vi "DerotatorControl_byYaw.vi"() -> ()   [LabVIEW 2021]
uses:
  <vilib>/DAQmx/write.llb/DAQmx Write (Digital Bool 1Line 1Point).vi
  <vilib>/DAQmx/create/channels.llb/DAQmx Create Channel (DO-Digital Output).vi
  <vilib>/DAQmx/miscellaneous.llb/DAQmx Fill In Error Info.vi
  GlobalYAW.vi
panel:
  out "Pitch":dbl(slide) scale=-90.0..90.0
  out "Roll":dbl(slide) scale=-180.0..180.0
  out "Yaw":dbl(slide) scale=-180.0..180.0
  in  "stop":bool
  in  "Record!":bool
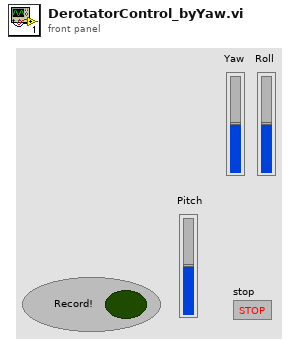
[diagram p1: front panel]
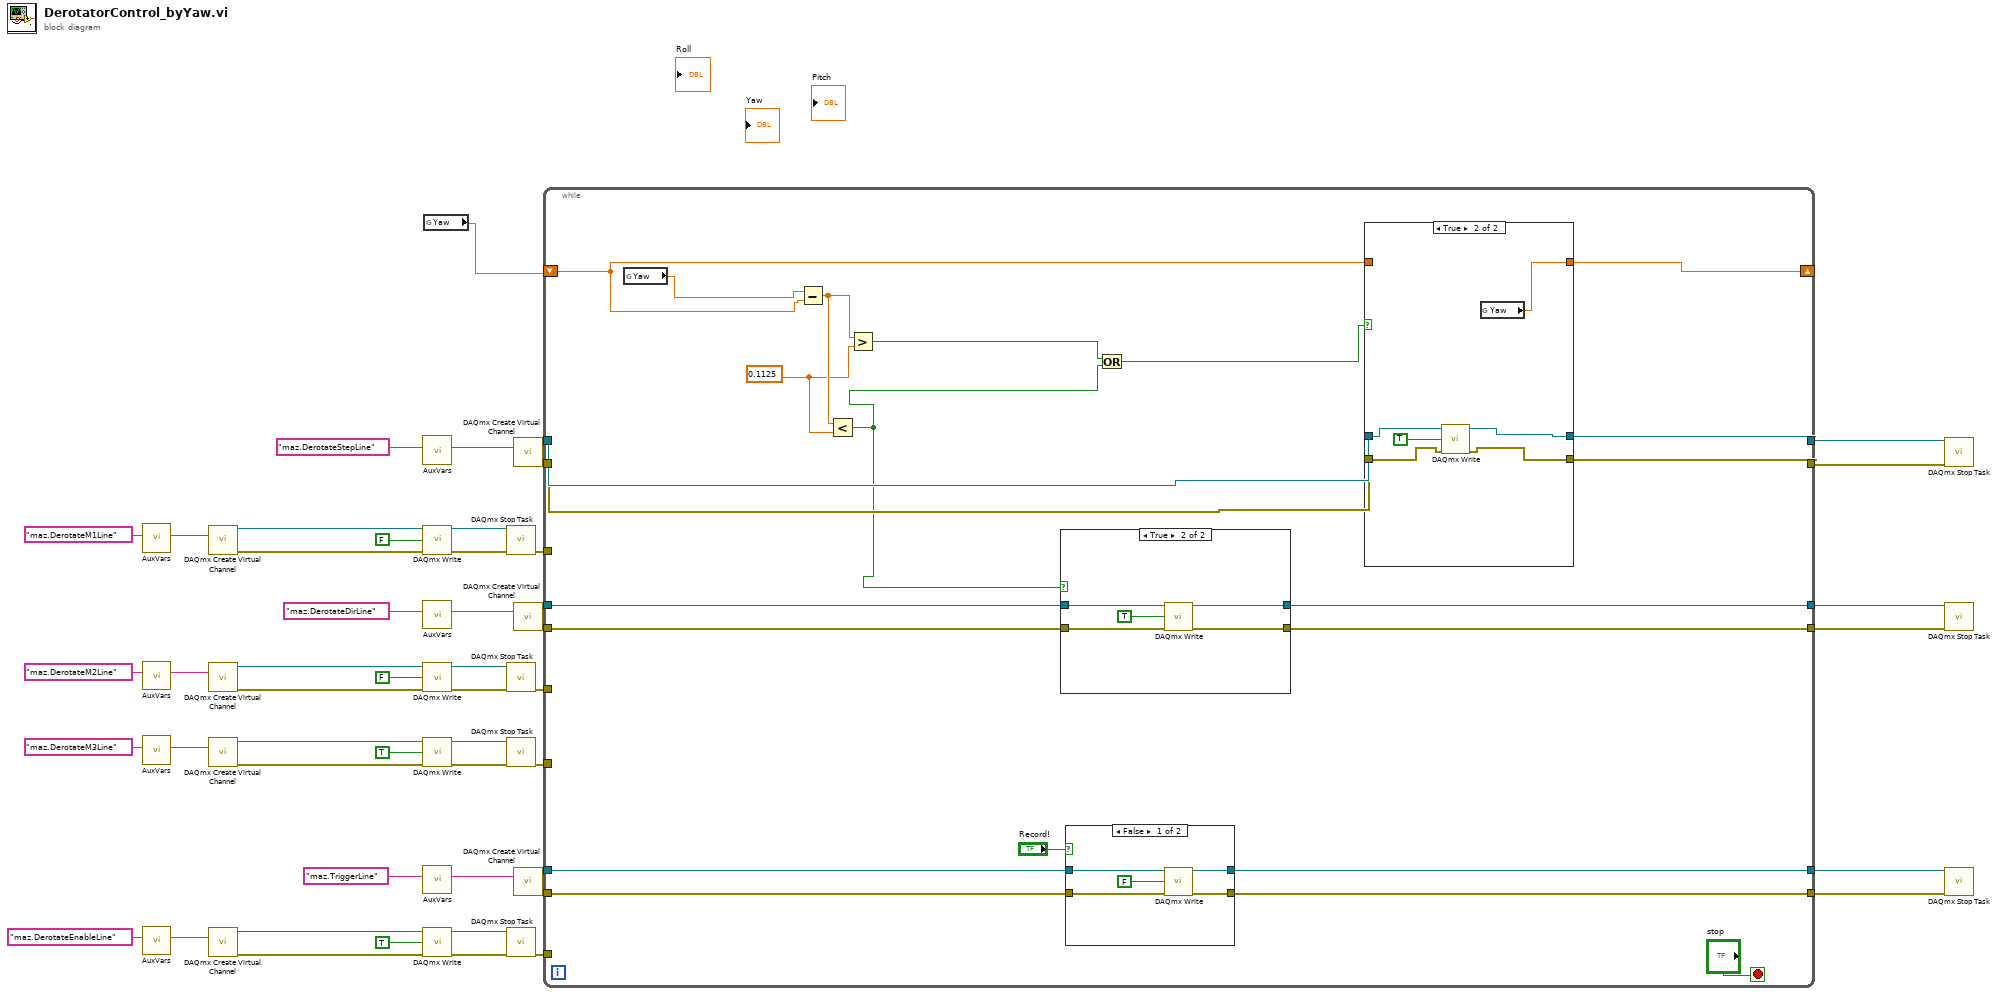
[diagram p0: block diagram]
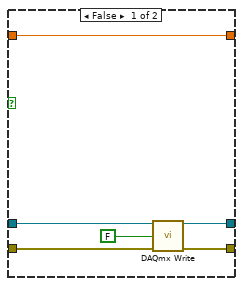
[diagram p2: hidden frame]
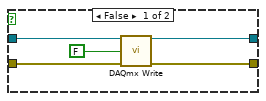
[diagram p3: hidden frame]
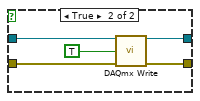
[diagram p4: hidden frame]
diagram:
  n1 = call "AuxVars.vi"("key"="maz.DerotateM1Line") -> ("value"=w26:string)  [unwired: 9 in, 1 out]
  n2 = call "AuxVars.vi"("key"="maz.DerotateM2Line") -> ("value"=w19:string)  [unwired: 9 in, 1 out]
  n3 = call "AuxVars.vi"("key"="maz.DerotateM3Line") -> ("value"=w12:string)  [unwired: 9 in, 1 out]
  n4 = call "AuxVars.vi"("key"="maz.DerotateEnableLine") -> ("value"=w41:string)  [unwired: 9 in, 1 out]
  n5 = call-poly <vilib>:"DAQmx Create Virtual Channel.vi"("lines"=w26) -> ("task out"=w23:refnum<k21>, "error out"=w20:errorcluster)  [unwired: 13 in]
  n6 = call-poly <vilib>:"DAQmx Create Virtual Channel.vi"("lines"=w19) -> ("task out"=w16:refnum<k21>, "error out"=w13:errorcluster)  [unwired: 13 in]
  n7 = call-poly <vilib>:"DAQmx Create Virtual Channel.vi"("lines"=w12) -> ("task out"=w9:refnum<k21>, "error out"=w6:errorcluster)  [unwired: 13 in]
  n8 = call-poly <vilib>:"DAQmx Create Virtual Channel.vi"("lines"=w41) -> ("task out"=w30:refnum<k21>, "error out"=w27:errorcluster)  [unwired: 13 in]
  n9 = call "AuxVars.vi"("key"="maz.DerotateStepLine") -> ("value"=w43:string)  [unwired: 9 in, 1 out]
  n10 = call-poly <vilib>:"DAQmx Write.vi"("task/channels in"=w23, "data"=FALSE, "error in"=w20) -> ("task out"=w22:refnum<k21>, "error out"=w21:errorcluster)  [unwired: 10 in, 1 out]
  n11 = call "AuxVars.vi"("key"="maz.DerotateDirLine") -> ("value"=w45:string)  [unwired: 9 in, 1 out]
  n12 = call-poly <vilib>:"DAQmx Write.vi"("task/channels in"=w16, "data"=FALSE, "error in"=w13) -> ("task out"=w15:refnum<k21>, "error out"=w14:errorcluster)  [unwired: 10 in, 1 out]
  n13 = call-poly <vilib>:"DAQmx Write.vi"("task/channels in"=w9, "data"=TRUE, "error in"=w6) -> ("task out"=w8:refnum<k21>, "error out"=w7:errorcluster)  [unwired: 10 in, 1 out]
  n14 = call "AuxVars.vi"("key"="maz.TriggerLine") -> ("value"=w51:string)  [unwired: 9 in, 1 out]
  n15 = call-poly <vilib>:"DAQmx Write.vi"("task/channels in"=w30, "data"=TRUE, "error in"=w27) -> ("task out"=w29:refnum<k21>, "error out"=w28:errorcluster)  [unwired: 10 in, 1 out]
  n16 = global read "GlobalYAW.vi" "Yaw"() -> (w1:dbl)
  n17 = call <vilib>:"DAQmx Stop Task.vi"("task/channels in"=w22, "error in"=w21) -> ("error out"=w4:errorcluster)  [unwired: 12 in, 1 out]
  n18 = call <vilib>:"DAQmx Stop Task.vi"("task/channels in"=w15, "error in"=w14) -> ("error out"=w3:errorcluster)  [unwired: 12 in, 1 out]
  n19 = call <vilib>:"DAQmx Stop Task.vi"("task/channels in"=w8, "error in"=w7) -> ("error out"=w2:errorcluster)  [unwired: 12 in, 1 out]
  n20 = call <vilib>:"DAQmx Stop Task.vi"("task/channels in"=w29, "error in"=w28) -> ("error out"=w5:errorcluster)  [unwired: 12 in, 1 out]
  n21 = call-poly <vilib>:"DAQmx Create Virtual Channel.vi"("lines"=w43) -> ("task out"=w39:refnum<k21>, "error out"=w38:errorcluster)  [unwired: 13 in]
  n22 = call-poly <vilib>:"DAQmx Create Virtual Channel.vi"("lines"=w45) -> ("task out"=w35:refnum<k21>, "error out"=w34:errorcluster)  [unwired: 13 in]
  n23 = call-poly <vilib>:"DAQmx Create Virtual Channel.vi"("lines"=w51) -> ("task out"=w49:refnum<k21>, "error out"=w48:errorcluster)  [unwired: 13 in]
  n24 = while {
    tunnel: w49 -> [w73]
    tunnel: w48 -> [w72]
    tunnel: [w71] -> w47
    tunnel: [w70] -> w46
    tunnel: w39 -> [w67]
    tunnel: w38 -> [w66]
    tunnel: [w65] -> w37
    tunnel: [w64] -> w36
    tunnel: w35 -> [w63]
    tunnel: w34 -> [w62]
    tunnel: [w61] -> w33
    tunnel: [w60] -> w32
    tunnel: w5 -> [_]
    tunnel: w4 -> [_]
    tunnel: w3 -> [_]
    tunnel: w2 -> [_]
    shift-right: [w57] -> _
    shift-left: w1 -> [w56]
    stop <- "stop" stop-if-true
    w58 = 0.1125
    n25 = global read "GlobalYAW.vi" "Yaw"() -> (w52:dbl)
    n26 = Subtract(x=w52, y=w56) -> (x-y=w59:dbl)
    n27 = Less?(x=w59, y=w58) -> (x < y?=w53:bool)
    n28 = Greater?(x=w59, y=w58) -> (0:w54:bool)
    n29 = case shown="True" w53 {
      tunnel: w63 -> [w89 w95]
      tunnel: w62 -> [w88 w94]
      tunnel: [w87 w93] -> w60
      tunnel: [w86 w92] -> w61
      frame False {
        n30 = call-poly <vilib>:"DAQmx Write.vi"("task/channels in"=w89, "data"=FALSE, "error in"=w88) -> ("task out"=w87:refnum<k21>, "error out"=w86:errorcluster)  [unwired: 10 in, 1 out]
      }
      frame True {
        n31 = call-poly <vilib>:"DAQmx Write.vi"("task/channels in"=w95, "data"=TRUE, "error in"=w94) -> ("task out"=w93:refnum<k21>, "error out"=w92:errorcluster)  [unwired: 10 in, 1 out]
      }
    }
    n32 = case shown="False" "Record!" {
      tunnel: w73 -> [w99 w105]
      tunnel: w72 -> [w98 w104]
      tunnel: [w97 w103] -> w71
      tunnel: [w96 w102] -> w70
      frame False {
        n33 = call-poly <vilib>:"DAQmx Write.vi"("task/channels in"=w99, "data"=FALSE, "error in"=w98) -> ("task out"=w97:refnum<k21>, "error out"=w96:errorcluster)  [unwired: 10 in, 1 out]
      }
      frame True {
        n34 = call-poly <vilib>:"DAQmx Write.vi"("task/channels in"=w105, "data"=TRUE, "error in"=w104) -> ("task out"=w103:refnum<k21>, "error out"=w102:errorcluster)  [unwired: 10 in, 1 out]
      }
    }
    n35 = Or(x=w54, y=w53) -> (x .or. y?=w55:bool)
    n36 = case shown="True" w55 {
      tunnel: w67 -> [w78 w84]
      tunnel: w66 -> [w77 w83]
      tunnel: [w76 w81] -> w64
      tunnel: [w75 w82] -> w65
      tunnel: [w74 w80] -> w57
      tunnel: w56 -> [w74 _]
      frame False {
        n37 = call-poly <vilib>:"DAQmx Write.vi"("task/channels in"=w78, "data"=FALSE, "error in"=w77) -> ("task out"=w76:refnum<k21>, "error out"=w75:errorcluster)  [unwired: 10 in, 1 out]
      }
      frame True {
        n38 = call-poly <vilib>:"DAQmx Write.vi"("task/channels in"=w84, "data"=TRUE, "error in"=w83) -> ("task out"=w81:refnum<k21>, "error out"=w82:errorcluster)  [unwired: 10 in, 1 out]
        n39 = global read "GlobalYAW.vi" "Yaw"() -> (w80:dbl)
      }
    }
  }
  n40 = call <vilib>:"DAQmx Stop Task.vi"("task/channels in"=w36, "error in"=w37) -> ()  [unwired: 12 in, 2 out]
  n41 = call <vilib>:"DAQmx Stop Task.vi"("task/channels in"=w32, "error in"=w33) -> ()  [unwired: 12 in, 2 out]
  n42 = call <vilib>:"DAQmx Stop Task.vi"("task/channels in"=w47, "error in"=w46) -> ()  [unwired: 12 in, 2 out]
